vi "Esercitazione 5 - Incertezza di categoria A.vi"() -> ()   [LabVIEW 2021]
panel:
  out "Valore relativo incertezza (%)":dbl
  out "Incertezza assoluta":dbl format="%#_6f"
  out "Scarto sperimentale":dbl format="%#_6f"
  out "Array":dbl[](array[numeric])
  out "Miglior stima del misurando":dbl
  out "sum":dbl
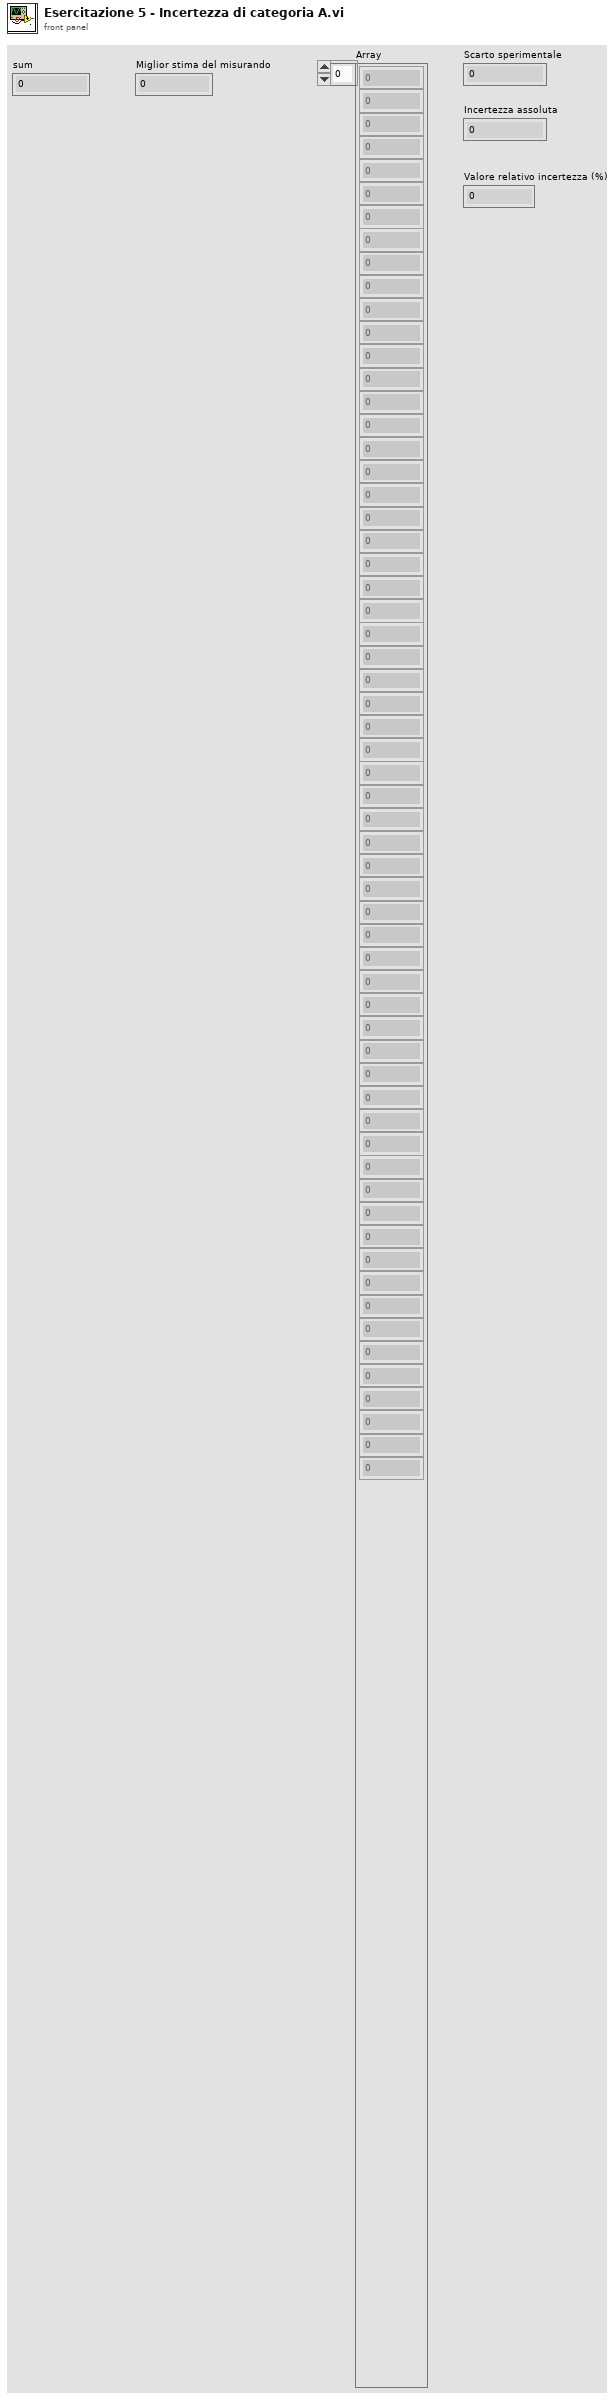
[diagram p1: front panel]
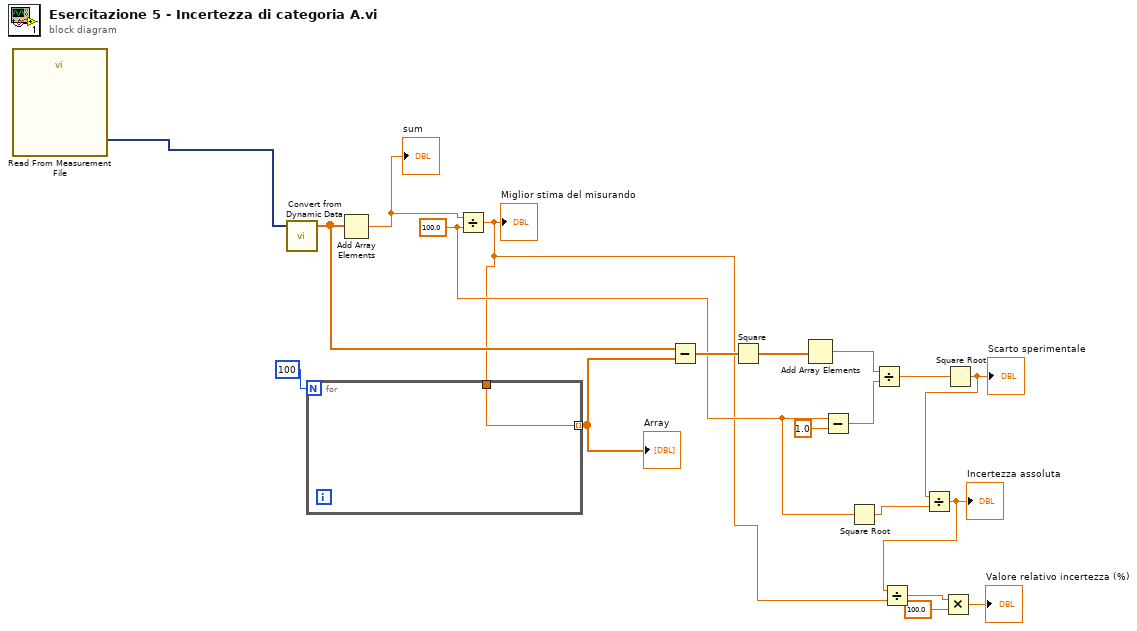
[diagram p0: block diagram]
diagram:
  w7 = 100.0 ("y")
  n1 = call "Read From Measurement File"() -> ("Signals"=w1:dynamicdata)  [unwired: 6 in, 5 out]
  n2 = call "Convert from Dynamic Data"("Dynamic Data Type"=w1) -> ("Array"=w15:dbl[])  [unwired: 3 in]
  n3 = Add Array Elements(numeric array=w15) -> (sum=w19:dbl)
  "sum" <- w19
  n4 = Divide(x=w19, y=w7) -> (x/y=w5:dbl)
  "Miglior stima del misurando" <- w5
  n5 = for {
    N: 100 -> [_]
    tunnel: w5 -> [w20]
    tunnel: [w20] -> w17 mode=indexing
  }
  "Array" <- w17
  n6 = Subtract(x=w15, y=w17) -> (x-y=w16:dbl[])
  n7 = Square(x=w16) -> (x^2=w14:dbl[])
  n8 = Add Array Elements(numeric array=w14) -> (sum=w13:dbl)
  n9 = Subtract(x=w7, y=1.0) -> (x-y=w10:dbl)
  n10 = Square Root(x=w7) -> (sqrt(x)=w8:dbl)
  n11 = Divide(x=w13, y=w10) -> (x/y=w12:dbl)
  n12 = Square Root(x=w12) -> (sqrt(x)=w11:dbl)
  "Scarto sperimentale" <- w11
  n13 = Divide(x=w11, y=w8) -> (x/y=w6:dbl)
  "Incertezza assoluta" <- w6
  n14 = Divide(x=w6, y=w5) -> (x/y=w4:dbl)
  n15 = Multiply(x=w4, y=100.0) -> (x*y=→"Valore relativo incertezza (%)":dbl)
